vi "FCI_Right_Cam_Coord.vi"(0 "Image In":T7(plugin-control), 1 "Search Direction":u32(ring) items=["Left to Right", "Right to Left", "Top to Bottom", "Bottom to Top"], 5 "ROI Descriptor":T1 {"Contours"."Type" items=["No Selection", "Point", "Line", "Rectangle", "Oval", "Polygon", "Free", "Annulus", "Unused2", "Unused3", "Broken Line", "Free Hand Line", "Rotated Rectangle"]}, 7 "Edge Options":T5={"Edge Polarity"=2, "Kernel Size"=3, "Width"=3, "Minimum Edge Strength"=50.0, "Interpolation Type"=enum."Zero Order", "Data Processing Method"=enum."Average"} {"Edge Polarity" items=["All Edges", "Rising Edges", "Falling Edges"]; "Minimum Edge Strength" format="%.2f"; "Width" step=2; "Kernel Size" step=2}, 9 "Line Options":T2={"Number of Lines"=1, "Type"=enum."First Edge Rake", "Min. Score"=10.0, "Max. Score"=1000.0, "Orientation"=0.0, "Angle Range"=80.0, "Angle Tolerance"=1.0, "Step Size"=18, "Min. SNR (db)"=0.0, "Min. Points (%)"=25.0, "Hough Iterations"=5} {"Min. Points (%)" min=0.0 max=100.0; "Min. SNR (db)" min=0.0; "Max. Score" min=0.0 max=1024.0; "Min. Score" min=0.0 max=1024.0 step=1.0}, 11 "error in (no error)":errorcluster) -> (4 "Coordinate System":T4 {"Axis Reference" items=["Direct", "Indirect"]; "Angle (deg)" format="%.2f"; "Origin"."Y" format="%.2f"; "Origin"."X" format="%.2f"}, 15 "error out":errorcluster)   [LabVIEW 2019, in "Algorithm.lvclass"]
uses:
  FrameworkOverrides/Algorithm.lvclass
  <vilib>/vision/NI_Vision_Development_Module.lvlib
  <vilib>/vision/Measure.llb/Edge Polarity.ctl
  <vilib>/vision/Measure.llb/Edge Options.ctl
  <vilib>/vision/Measure.llb/Straight Edge Process.ctl
  <vilib>/vision/Measure.llb/Straight Edge Options.ctl
panel:
  out "output cluster":T2={"Number of Lines"=1, "Type"=enum."Best Edge Projection", "Min. Score"=0.0, "Max. Score"=1000.0, "Orientation"=0.0, "Angle Range"=5.0, "Angle Tolerance"=0.0, "Step Size"=5, "Min. SNR (db)"=0.0, "Min. Points (%)"=25.0, "Hough Iterations"=5} {"Min. Points (%)" min=0.0 max=100.0; "Min. SNR (db)" min=0.0; "Max. Score" min=0.0 max=1024.0; "Min. Score" min=0.0 max=1024.0 step=1.0}
  out "Angle":dbl format="%.2f"
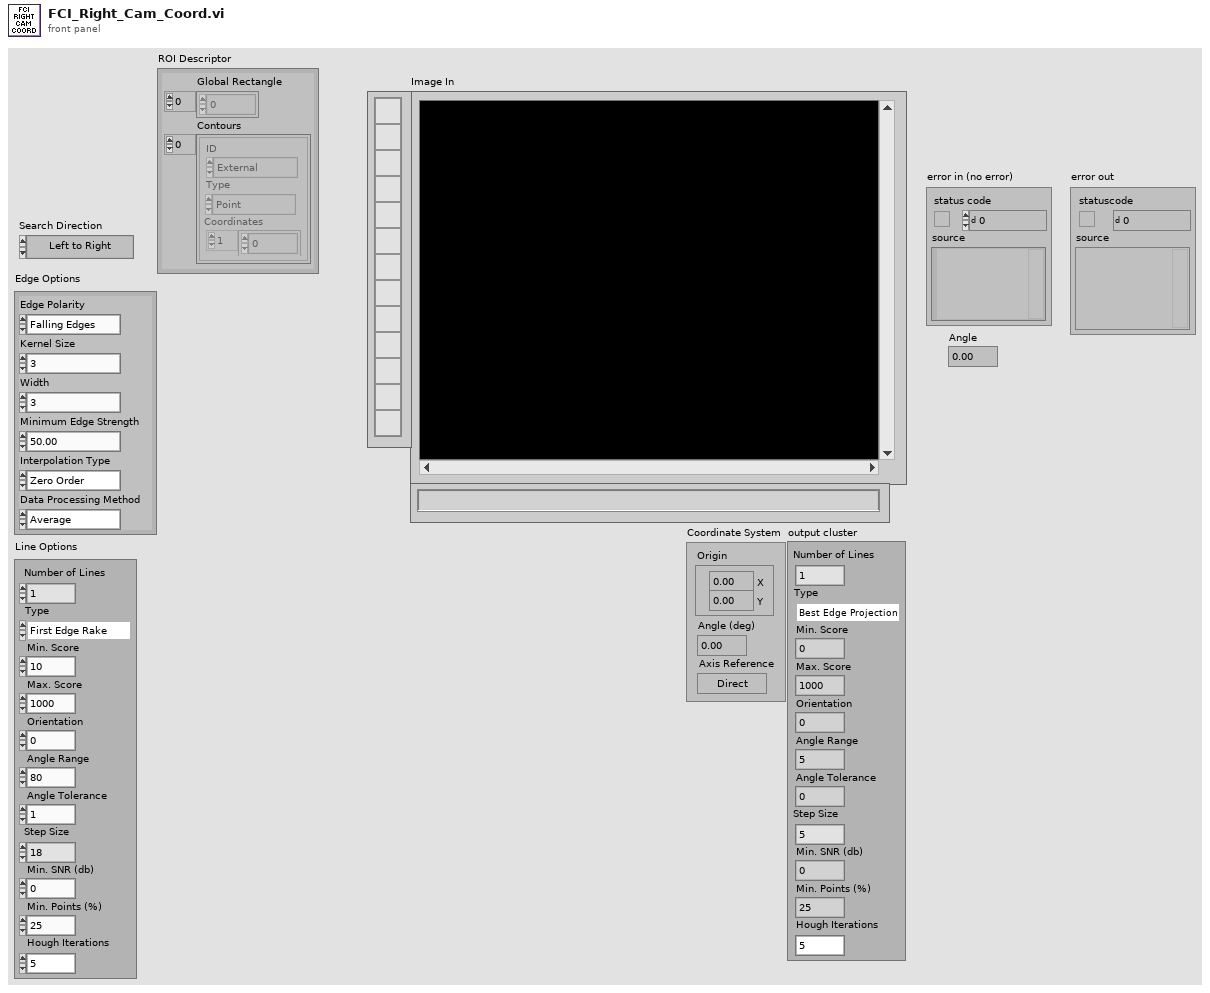
[diagram p1: front panel]
types:
  T1 = cluster{"Global Rectangle":i32[], "Contours":cluster{"ID":enum32{"External", "Internal"}, "Type":u32, "Coordinates":i32[]}[]}
  T2 = typedef "Straight Edge Options.ctl" = cluster{"Number of Lines":i32, "Type":T3, "Min. Score":dbl, "Max. Score":dbl, "Orientation":dbl, "Angle Range":dbl, "Angle Tolerance":dbl, "Step Size":u32, "Min. SNR (db)":dbl, "Min. Points (%)":dbl, "Hough Iterations":i32}
  T3 = typedef "Straight Edge Process.ctl" = enum32{"First Edge Rake", "Best Edge Rake", "Hough Edge Rake", "First Edge Projection", "Best Edge Projection"}
  T4 = cluster{"Origin":cluster{"X":sgl, "Y":sgl}, "Angle (deg)":sgl, "Axis Reference":u32}
  T5 = typedef "Edge Options.ctl" = cluster{"Edge Polarity":T6, "Kernel Size":u32, "Width":u32, "Minimum Edge Strength":sgl, "Interpolation Type":enum32{"Zero Order", "Bilinear", "Quadratic", "Cubic", "Bilinear Fixed"}, "Data Processing Method":enum32{"Average", "Median"}}
  T6 = typedef "Edge Polarity.ctl" = u32
  T7 = typedef "IMAQ Image.ctl" = refnum<image>
  T8 = cluster{"Point1 (Pixels)":cluster{"X":sgl, "Y":sgl}, "Point2 (Pixels)":cluster{"X":sgl, "Y":sgl}, "Point1 (Real-World)":cluster{"X":sgl, "Y":sgl}, "Point2 (Real-World)":cluster{"X":sgl, "Y":sgl}, "Angle (Pixel)":dbl, "Angle (Real-World)":dbl, "Score":dbl, "Straightness":dbl, "Average SNR (db)":dbl, "Calibration Valid":bool}[]
  T9 = typedef "Search Line.ctl" = cluster{"Start Point":cluster{"X":sgl, "Y":sgl}, "End Point":cluster{"X":sgl, "Y":sgl}, "Edge Info":T10[], "Edge Map":dbl[], "Calibration Valid":bool}
  T10 = typedef "Edge New.ctl" = cluster{"Location (Pixel)":cluster{"X":sgl, "Y":sgl}, "Location (Real-World)":cluster{"X":sgl, "Y":sgl}, "Distance (Pixel)":dbl, "Distance (Real-World)":dbl, "Strength":dbl, "Noise":dbl, "Rising?":bool}
  T11 = cluster{"Point1 (Pixels)":cluster{"X":sgl, "Y":sgl}, "Point2 (Pixels)":cluster{"X":sgl, "Y":sgl}, "Point1 (Real-World)":cluster{"X":sgl, "Y":sgl}, "Point2 (Real-World)":cluster{"X":sgl, "Y":sgl}, "Angle (Pixel)":dbl, "Angle (Real-World)":dbl, "Score":dbl, "Straightness":dbl, "Average SNR (db)":dbl, "Calibration Valid":bool}
  T12 = cluster{"Point1 (Pixels)":cluster{"X":sgl, "Y":sgl}, "Point2 (Pixels)":cluster{"X":sgl, "Y":sgl}}
  T13 = cluster{"Intersection Point":cluster{"X":sgl, "Y":sgl}}
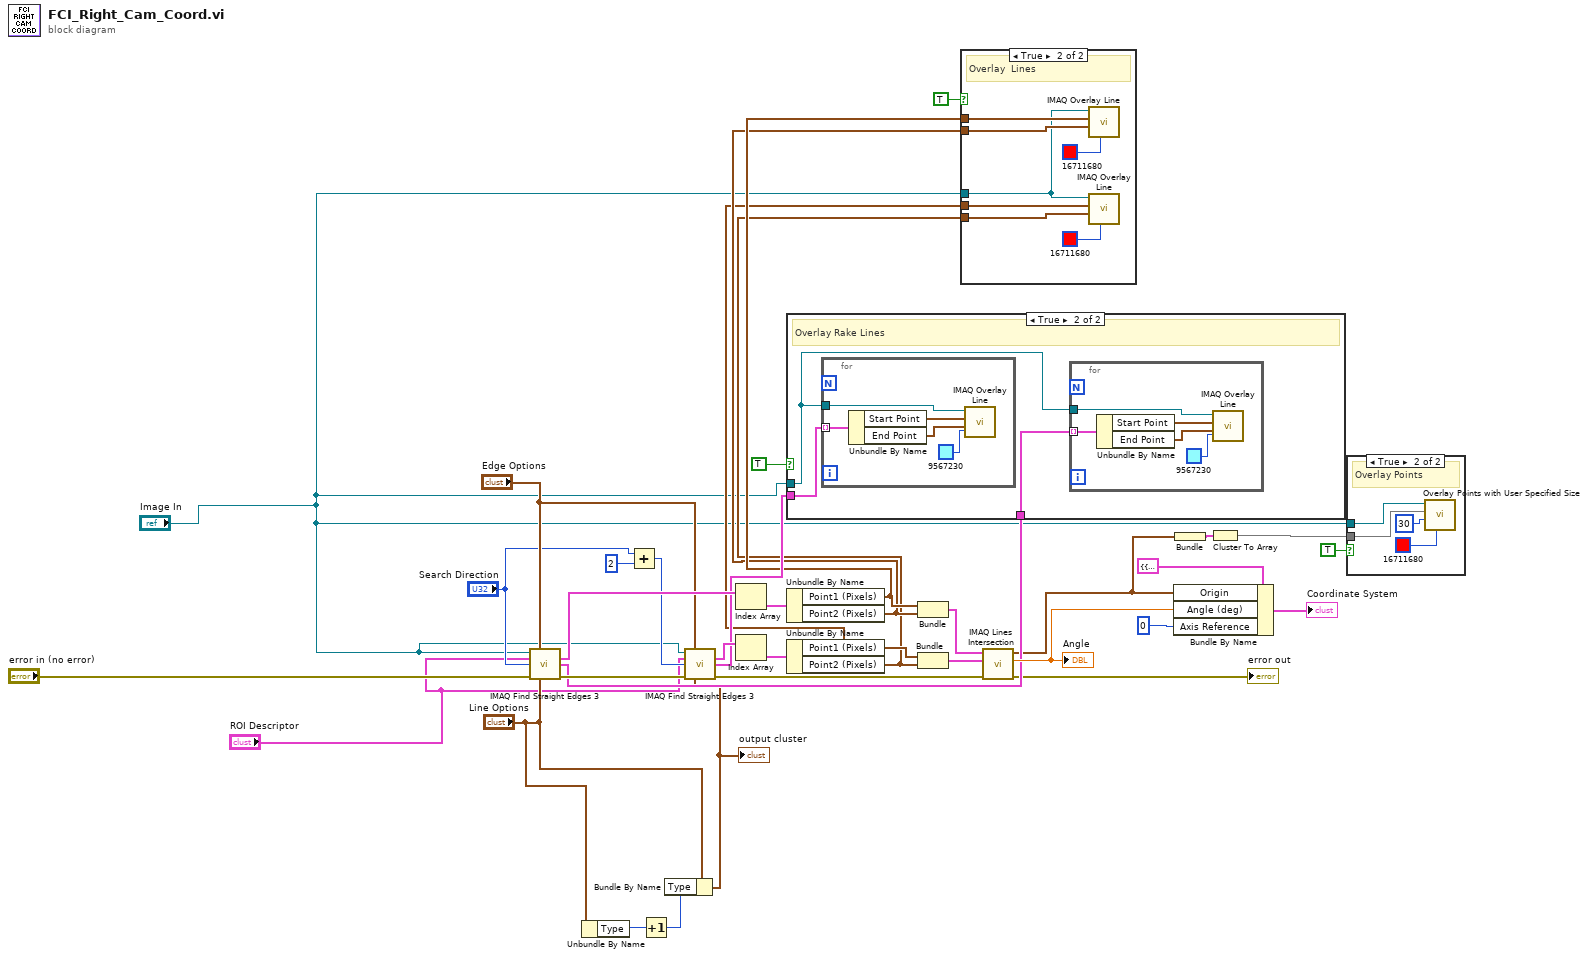
[diagram p0: block diagram]
diagram:
  n1 = call "IMAQ Find Straight Edges 3"("Image"="Image In", "Edge Options"="Edge Options", "ROI Descriptor"="ROI Descriptor", "Search Direction"="Search Direction", "error in (no error)"="error in (no error)", "Line Options"="Line Options") -> ("Straight Edges"=w34:T8, "Search Lines Information"=w16:T9[], "error out"=w24:errorcluster)  [unwired: 5 in, 2 out]
  n2 = Unbundle By Name("Line Options") -> ("Type"=w13:T3)
  n3 = Add(x="Search Direction", y=u32 2) -> (x+y=w7:u32)
  n4 = Increment(x=w13) -> (x+1=w12:T3)
  n5 = Bundle By Name(cluster="Line Options", "Type"=w12) -> (w11:T2)
  "output cluster" <- w11
  n6 = call "IMAQ Find Straight Edges 3"("Image"="Image In", "Edge Options"="Edge Options", "ROI Descriptor"="ROI Descriptor", "Search Direction"=w7, "error in (no error)"=w24, "Line Options"=w11) -> ("Straight Edges"=w36:T8, "Search Lines Information"=w30:T9[], "error out"=w19:errorcluster)  [unwired: 5 in, 2 out]
  n7 = Index Array(array=w34) -> (element=w33:T11)  [unwired: 1 in]
  n8 = Index Array(array=w36) -> (element=w35:T11)  [unwired: 1 in]
  n9 = case shown="True" TRUE {
    tunnel: w30 -> [_ w39]
    tunnel: "Image In" -> [_ w37]
    tunnel: w16 -> [_ w38]
    frame False {
    }
    frame True {
      # "Overlay Rake Lines"
      n10 = for {
        tunnel: w39 -> [w49] mode=indexing
        tunnel: w37 -> [w46]
        n11 = Unbundle By Name(w49) -> ("Start Point"=w48:cluster{"X":sgl, "Y":sgl}, "End Point"=w47:cluster{"X":sgl, "Y":sgl})
        n12 = call "IMAQ Overlay Line"("Color"=u32 9567230, "End Point"=w47, "Start Point"=w48, "Image"=w46) -> ()  [unwired: 6 in, 2 out]
      }
      n13 = for {
        tunnel: w38 -> [w44] mode=indexing
        tunnel: w37 -> [w41]
        n14 = Unbundle By Name(w44) -> ("Start Point"=w43:cluster{"X":sgl, "Y":sgl}, "End Point"=w42:cluster{"X":sgl, "Y":sgl})
        n15 = call "IMAQ Overlay Line"("Color"=u32 9567230, "End Point"=w42, "Start Point"=w43, "Image"=w41) -> ()  [unwired: 6 in, 2 out]
      }
    }
  }
  n16 = Unbundle By Name(w33) -> ("Point1 (Pixels)"=w26:cluster{"X":sgl, "Y":sgl}, "Point2 (Pixels)"=w25:cluster{"X":sgl, "Y":sgl})
  n17 = Unbundle By Name(w35) -> ("Point1 (Pixels)"=w22:cluster{"X":sgl, "Y":sgl}, "Point2 (Pixels)"=w21:cluster{"X":sgl, "Y":sgl})
  n18 = Bundle("Point1 (Pixels)"=w26, "Point2 (Pixels)"=w25) -> (w23:T12)  [unwired: 1 in]
  n19 = Bundle("Point1 (Pixels)"=w22, "Point2 (Pixels)"=w21) -> (w20:T12)  [unwired: 1 in]
  n20 = case shown="True" TRUE {
    tunnel: "Image In" -> [_ w50]
    tunnel: w26 -> [_ w54]
    tunnel: w25 -> [_ w53]
    tunnel: w22 -> [_ w52]
    tunnel: w21 -> [_ w51]
    frame False {
    }
    frame True {
      # "Overlay  Lines"
      n21 = call "IMAQ Overlay Line"("Color"=u32 16711680, "End Point"=w53, "Start Point"=w54, "Image"=w50) -> ()  [unwired: 6 in, 2 out]
      n22 = call "IMAQ Overlay Line"("Color"=u32 16711680, "End Point"=w51, "Start Point"=w52, "Image"=w50) -> ()  [unwired: 6 in, 2 out]
    }
  }
  n23 = call "IMAQ Lines Intersection"("error in (no error)"=w19, "Line 2"=w20, "Line 1"=w23) -> ("error out"=→"error out":errorcluster, "Angle"=w18:dbl, "Intersection Point"=w3:cluster{"X":sgl, "Y":sgl})  [unwired: 6 in]
  "Angle" <- w18
  n24 = Bundle By Name(cluster=T4 {"Origin"={"X"=0.0, "Y"=0.0}, "Angle (deg)"=0.0, "Axis Reference"=0} ("Coordinate System"), "Origin"=w3, "Angle (deg)"=w18, "Axis Reference"=u32 0) -> (→"Coordinate System":T4)
  n25 = Bundle("Intersection Point"=w3) -> (w2:T13)  [unwired: 1 in]
  n26 = Cluster To Array(cluster=w2) -> (array=w1:cluster{"X":sgl, "Y":sgl}[])
  n27 = case shown="True" TRUE {
    tunnel: "Image In" -> [_ w58]
    tunnel: w1 -> [_ w57]
    frame False {
    }
    frame True {
      # "Overlay Points"
      n28 = call "Overlay Points with User Specified Size.vi"("Color"=u32 16711680, "Point Diameter (5)"=u32 30, "Points"=w57, "Image In"=w58) -> ()  [unwired: 6 in, 2 out]
    }
  }
